vi "GaiaActionWaitStateReady.vi"(8 "Error in":errorcluster, 9 "Timeout":i32, 10 "Application":string, 11 "ClientRef":refnum<k24>) -> (0 "error out":errorcluster, 3 "ClientRef out":refnum<k24>)   [LabVIEW 2018]
uses:
  C:/GIT/gaialabviewclient/Gaia_LabVIEW/Resources/JOT.GaiaClient.dll
  Gaia_LabVIEW/Resources/JOT.GaiaClient.dll
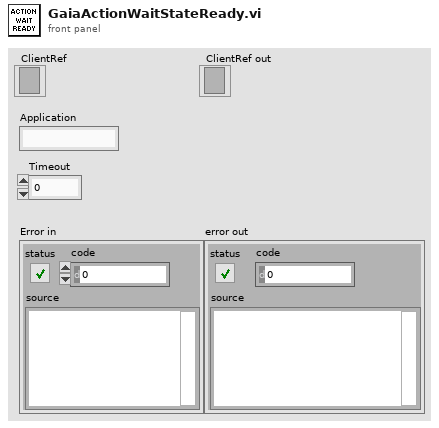
[diagram p1: front panel]
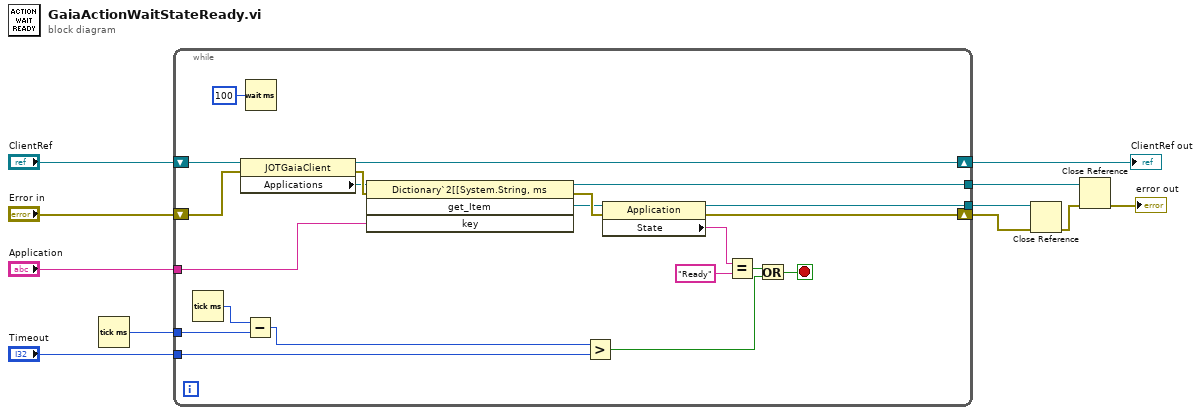
[diagram p0: block diagram]
diagram:
  n1 = Tick Count (ms)() -> (millisecond timer value=w1:u32)
  n2 = while {
    tunnel: "Application" -> [w28]
    shift-right: [w31] -> w11
    shift-left: "ClientRef" -> [w30]
    tunnel: [w25] -> w7
    tunnel: [w23] -> w5
    shift-right: [w24] -> w6
    shift-left: "Error in" -> [w22]
    tunnel: "Timeout" -> [w15]
    tunnel: w1 -> [w17]
    stop <- w12 stop-if-true
    n3 = Tick Count (ms)() -> (millisecond timer value=w18:u32)
    n4 = property class="JOTGaiaClient"(reference=w30, error in=w22) -> (reference out=w31:refnum<k24>, error out=w32:errorcluster, "Applications"=w29:refnum<k24>)
    n5 = Subtract(x=w18, y=w17) -> (x-y=w16:u32)
    n6 = Wait (ms)(milliseconds to wait=u32 100) -> ()  [unwired: 1 out]
    n7 = invoke class="Dictionary`2[[System.String, ms" method="get_Item"(reference=w29, error in=w32, "key"=w28) -> (reference out=w25:refnum<k24>, error out=w27:errorcluster, "get_Item"=w26:refnum<k24>)  [unwired: 1 in, 1 out]
    n8 = Greater?(x=w16, y=w15) -> (0:w13:bool)
    n9 = property class="Application"(reference=w26, error in=w27) -> (reference out=w23:refnum<k24>, error out=w24:errorcluster, "State"=w21:string)
    n10 = Equal?(x=w21, y="Ready" ("State")) -> (x = y?=w14:bool)
    n11 = Or(x=w14, y=w13) -> (x .or. y?=w12:bool)
  }
  "ClientRef out" <- w11
  n12 = Close Reference(reference=w5, error in (no error)=w6) -> (error out=w8:errorcluster)
  n13 = Close Reference(reference=w7, error in (no error)=w8) -> (error out=→"error out":errorcluster)
